vi "Read Config Section.vi"(8 "error in":errorcluster, 11 "Data in":T1) -> (0 "error out":errorcluster, 3 "Data out":T1)   [LabVIEW 2021, in "Main INI.lvlib"]
uses:
  Main INI.lvlib
  <vilib>/Utility/config.llb/NI_LVConfig.lvlib
  <userlib>/_OpenG.lib/variantconfig/variantconfig.llb/openg_variant_configuration_file.lvlib
  Core Data.ctl
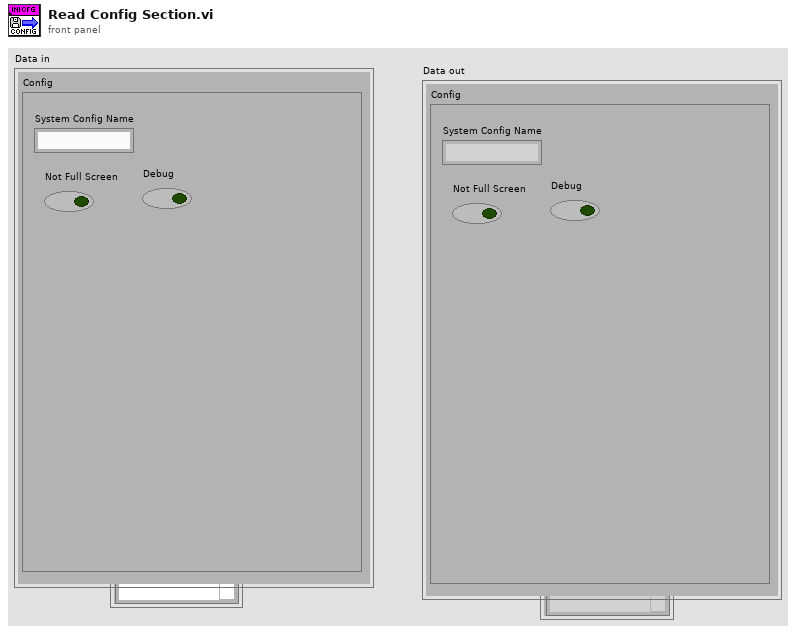
[diagram p1: front panel]
types:
  T1 = typedef "Main INI.lvlib/Core Data.ctl" = cluster{"Config":cluster{"System Config Name":string, "Not Full Screen":bool, "Debug":bool}}
  T2 = cluster{"System Config Name":string, "Not Full Screen":bool, "Debug":bool}
  T3 = typedef "NI_LVConfig.lvlib/Config Data RefNum.ctl" = refnum<k1>
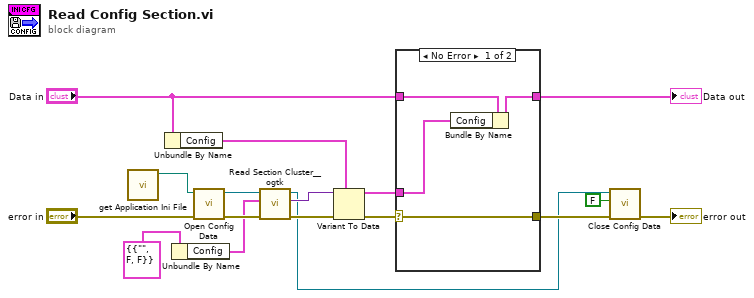
[diagram p0: block diagram]
diagram:
  n1 = call "get Application Ini File.vi"() -> ("Application Ini File"=w4:path)  [unwired: 11 in]
  n2 = Unbundle By Name("Data in") -> ("Config"=w3:T2)
  n3 = Unbundle By Name(T1 {"Config"={"System Config Name"="", "Not Full Screen"=FALSE, "Debug"=FALSE}} ("LV2 Data")) -> ("Config"=w1:T2)
  n4 = call <vilib>:"Open Config Data.vi"("error in (no error)"="error in", "configuration file path"=w4) -> ("error out"=w13:errorcluster, "refnum"=w12:T3)  [unwired: 7 in, 1 out]
  n5 = call <userlib>:"Read Section Cluster__ogtk.vi"("error in (no error)"=w13, "Section Formatted Cluster Type"=w1, "refnum"=w12) -> ("error out"=w14:errorcluster, "Section Formatted Cluster"=w9:variant, "dup refnum"=w5:T3)  [unwired: 4 in, 2 out]
  n6 = Variant To Data(error in=w14, type=w3, Variant=w9) -> (data=w8:T2, error out=w11:errorcluster)
  n7 = case shown="No Error" w11 {
    selector: w11 -> [w19 w22]
    tunnel: "Data in" -> [w21 w23]
    tunnel: w8 -> [w20 _]
    tunnel: [w19 w22] -> w7
    tunnel: [w18 w23] -> w6
    frame No Error {
      n8 = Bundle By Name(cluster=w21, "Config"=w20) -> (w18:T1)
    }
    frame Error {
    }
  }
  "Data out" <- w6
  n9 = call <vilib>:"Close Config Data.vi"("error in (no error)"=w7, "write file if changed (T)"=FALSE, "refnum"=w5) -> ("error out"=→"error out":errorcluster)  [unwired: 7 in, 1 out]
